vi "Compass.vi"(7 "GPS/Mag":bool, 8 "error in (no error)":errorcluster caption="Fehler (Eingang, kein Fehler)", 10 "MultiWii Data Cluster":T1 {"Altitude abs [m]" format="%.2f"; "Baro T [°C]" format="%.1f"; "Baro P [mbara]" format="%.1f"; "GPS_coord[LON]" format="%#_9f"; "GPS_coord[LAT]" format="%#_9f"; "Altitude [m]" format="%.2f"}) -> (0 "error out":errorcluster caption="Fehler (Ausgang)", 2 "Heading Digital":dbl format="%.1f", 3 "CompassGauge":picture)   [LabVIEW 2017]
uses:
  IMU_Functions/IMU_Data_Cluster.ctl
  <vilib>/Utility/miscctls.llb/LVBoundsTypeDef.ctl
  <vilib>/picture/picture.llb/imagedata.ctl
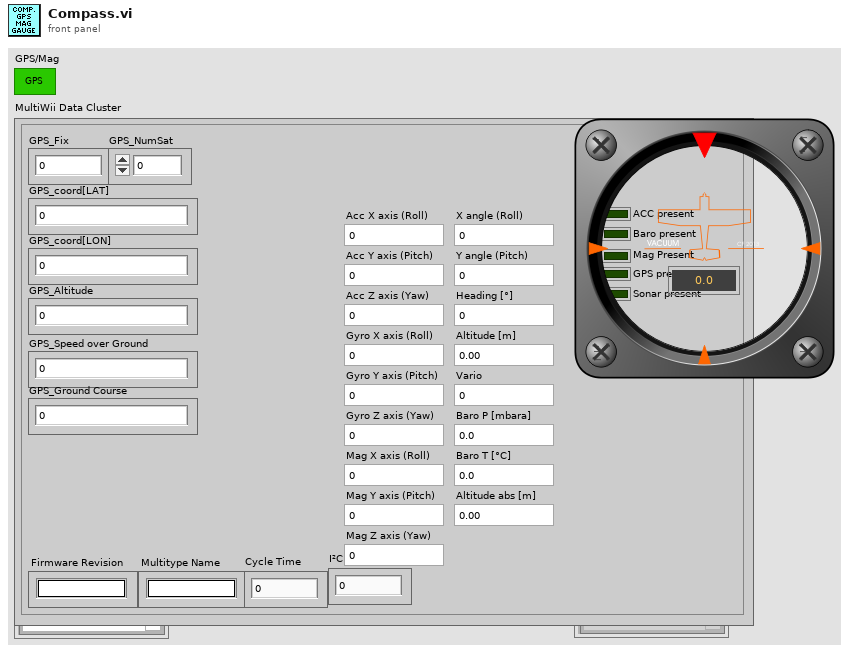
[diagram p1: front panel]
types:
  T1 = typedef "IMU_Data_Cluster.ctl" = cluster{"Firmware Revision":string, "Multitype Name":string, "Cycle Time":u16, "I²C Error Count":u16, "ACC present":bool, "Baro present":bool, "Mag Present":bool, "GPS present":bool, "Sonar present":bool, "Acc X axis (Roll)":dbl, "Acc Y axis (Pitch)":dbl, "Acc Z axis (Yaw)":dbl, "Gyro X axis (Roll)":dbl, "Gyro Y axis (Pitch)":dbl, "Gyro Z axis (Yaw)":dbl, "Mag X axis (Roll)":dbl, "Mag Y axis (Pitch)":dbl, "Mag Z axis (Yaw)":dbl, "X angle (Roll)":dbl, "Y angle (Pitch)":dbl, "Heading [°]":dbl, "Altitude [m]":dbl, "Vario":dbl, "GPS_Fix":u8, "GPS_NumSat":u8, "GPS_coord[LAT]":dbl, "GPS_coord[LON]":dbl, "GPS_Altitude":dbl, "GPS_Speed over Ground":dbl, "GPS_Ground Course":dbl, "Baro P [mbara]":dbl, "Baro T [°C]":dbl, "Altitude abs [m]":dbl}
  T2 = typedef "LVBoundsTypeDef.ctl" = cluster{"Width":u32, "Height":u32}
  T3 = typedef "imagedata.ctl" = cluster{"image type":i32, "image depth":i32, "image":u8[], "mask":u8[], "colors":u32[], "Rectangle":cluster{"left":i16, "top":i16, "right":i16, "bottom":i16}}
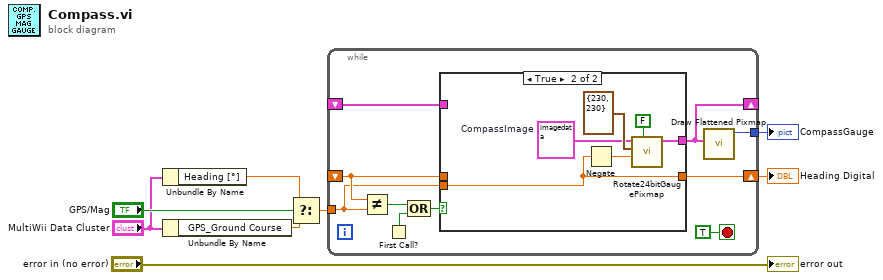
[diagram p0: block diagram]
diagram:
  n1 = Unbundle By Name("MultiWii Data Cluster") -> ("Heading [°]"=w8:dbl)
  n2 = Unbundle By Name("MultiWii Data Cluster") -> ("GPS_Ground Course"=w7:dbl)
  n3 = Select(t=w8, s="GPS/Mag", f=w7) -> (s? t:f=w1:dbl)
  n4 = while {
    shift-right: [w15] -> w3
    shift-left: _ -> [w14]
    tunnel: w1 -> [w9]
    shift-right: [w13] -> _
    shift-left: _ -> [w12]
    tunnel: [w10] -> w2
    stop <- TRUE stop-if-true
    n5 = Not Equal?(x=w14, y=w9) -> (x != y?=w16:bool)
    n6 = First Call?() -> (First Call?: T/F=w17:bool)
    n7 = Compound Arithmetic op=OR(w16, w17) -> (w18:bool)
    n8 = case shown="True" w18 {
      tunnel: [w20 w26] -> w13
      tunnel: w12 -> [w20 _]
      tunnel: w14 -> [w19 _]
      tunnel: [w19 w21] -> w15
      tunnel: w9 -> [_ w21]
      frame False {
      }
      frame True {
        w23 = T3 {"image type"=0, "image depth"=24, "image"=array[158700 elements], "mask"=[], "colors"=[], "Rectangle"={"left"=0, "top"=0, "right"=230, "bottom"=230}}  # CompassImage
        n9 = Negate(x=w21) -> (-x=w22:dbl)
        n10 = call "Rotate24bitGaugePixmap.vi"("Maske kombinieren? (F)"=FALSE, "Rotation Angle (degrees)"=w22, "Größe des Darstellungsbereichs"=T2 {"Width"=230, "Height"=230}, "image data"=w23) -> ("image data out"=w26:T3)  [unwired: 7 in]
      }
    }
    n11 = call <vilib>:"Draw Flattened Pixmap.vi"("image data"=w13) -> ("new picture"=w10:picture)  [unwired: 1 in, 7 out]
  }
  "Heading Digital" <- w3
  "CompassGauge" <- w2
  "error out" <- "error in (no error)"
